vi "Google Earth.vi"() -> ()   [LabVIEW 2011]
uses:
  SubVIs/EventHandlerEnum.ctl
panel:
  in  "Tab Control":enum32{"Main", "Debug Data"}(tab)
  in  "Tilt":dbl=70.0
  in  "FPV View":bool
  in  "stop?":bool
  in  "WebBrowser":refnum<k7>(container)
  out "StreamingProgressPercentage":i32(slide) scale=0.0..100.0
  out "Camera Position 2":T1
  out "Version":string
  out "VersionAppType":i32(ring) items=["EnterpriseClientGE"=0, "ProGE"=1, "PlusGE"=2, "FreeGE"=5, "UnknownGE"=255]
  out "ElevationExaggeration":dbl
  in  "Set":bool
  in  "AutoPilotSpeed":dbl=0.5
  in  "Camera Position":T2={"Azimuth"=0.0, "FocusPointAltitude"=0.0, "altMode"=1, "FocusPointLatitude"=0.0, "FocusPointLongitude"=0.0, "Range"=0.0, "Tilt"=0.0} {"altMode" items=["RelativeToGroundAltitudeGE"=1, "AbsoluteAltitudeGE"=2]}
  in  "EARTHLib.IApplicationGE 2":refnum<k7>
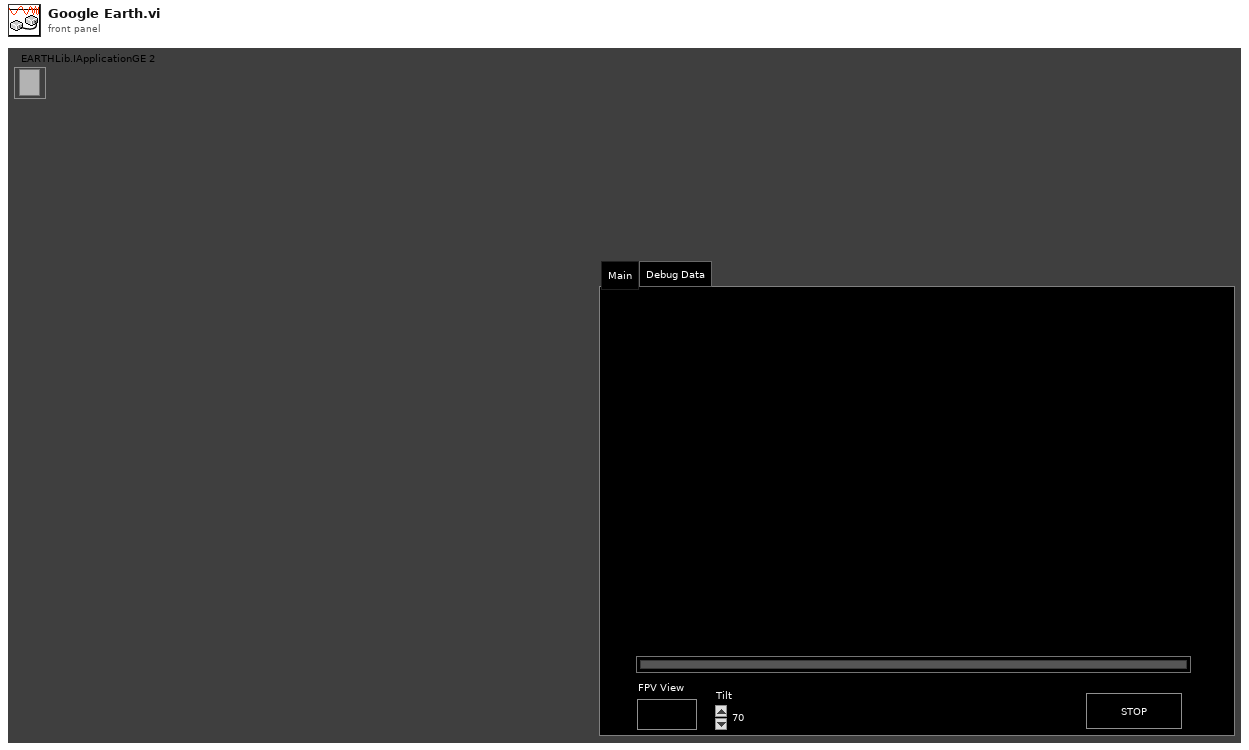
[diagram p1: front panel]
types:
  T1 = cluster{"Azimuth":dbl, "FocusPointAltitude":dbl, "FocusPointAltitudeMode":i32, "FocusPointLatitude":dbl, "FocusPointLongitude":dbl, "Range":dbl, "Tilt":dbl}
  T2 = cluster{"Azimuth":dbl, "FocusPointAltitude":dbl, "altMode":i32, "FocusPointLatitude":dbl, "FocusPointLongitude":dbl, "Range":dbl, "Tilt":dbl}
  T3 = typedef "EventHandlerEnum.ctl" = enum16{"Timeout", "Stop", "UpdateGEView", "FPV_View_On"}
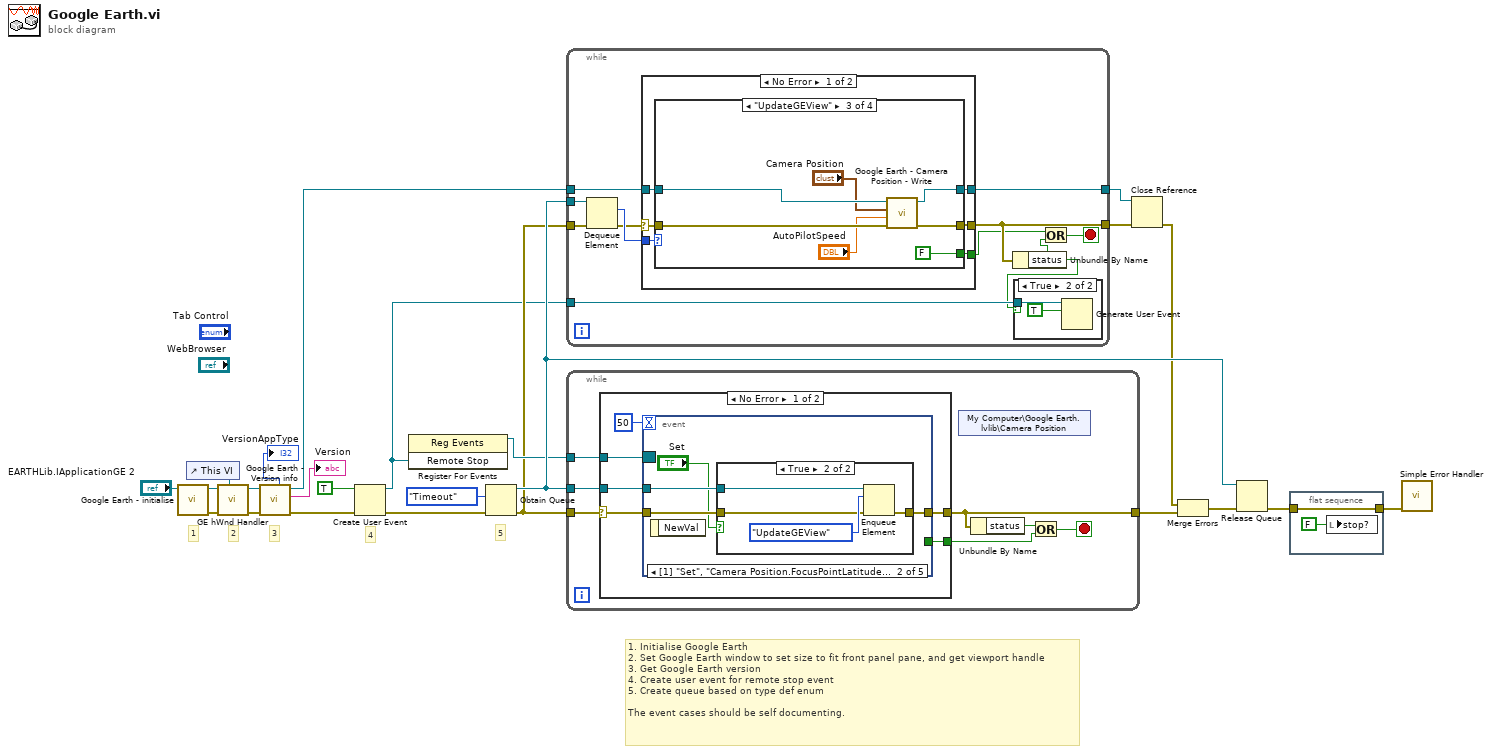
[diagram p0: block diagram]
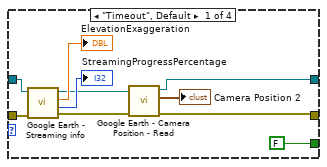
[diagram p3: hidden frame]
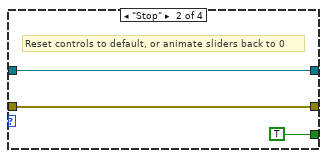
[diagram p4: hidden frame]
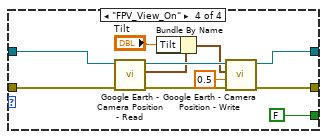
[diagram p5: hidden frame]
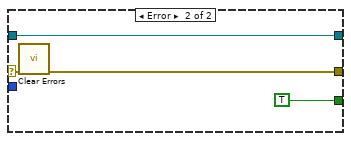
[diagram p6: hidden frame]
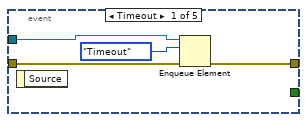
[diagram p7: hidden frame]
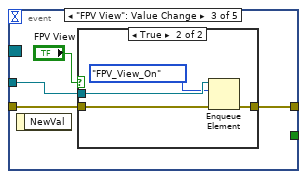
[diagram p9: hidden frame]
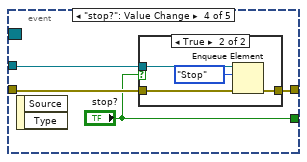
[diagram p11: hidden frame]
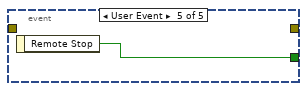
[diagram p13: hidden frame]
diagram:
  # "1. Initialise Google Earth\n2. Set Google Earth window to set size to fit front panel pane, and get viewport handle\n3. Get Google Earth version\n4. Create user event for remote stop event\n5. Create queue based on type def enum\n\nThe event cases should be self documenting."
  # "5"
  # "4"
  # "3"
  # "2"
  # "1"
  n1 = call "Google Earth - initialise.vi"("EARTHLib.IApplicationGE"="EARTHLib.IApplicationGE 2") -> ("error out"=w14:errorcluster, "Refnum Out"=w13:refnum<k7>)  [unwired: 8 in, 1 out]
  n2 = control-ref of="This VI"() -> (w21:refnum<vi>)
  n3 = call "GE hWnd Handler.vi"("This VI"=w21, "error in"=w14, "Refnum In"=w13) -> ("error out"=w22:errorcluster, "Refnum Out"=w15:refnum<k7>)  [unwired: 7 in]
  n4 = call "Google Earth - Version info.vi"("error in"=w22, "Refnum In"=w15) -> ("error out"=w2:errorcluster, "Version"=→"Version":string, "Refnum Out"=w19:refnum<k7>, "VersionAppType"=→"VersionAppType":i32)  [unwired: 6 in]
  n5 = Create User Event(user event datatype=TRUE ("Remote Stop"), error in=w2) -> (user event=w8:refnum<user-event>, error out=w12:errorcluster)
  n6 = register-events(w8) -> (reference out=w11:refnum<event-registration>)  [unwired: 2 in, 1 out]
  n7 = Obtain Queue(element data type=EventHandlerEnum."Timeout" ("Enum"), error in (no error)=w12) -> (queue out=w23:refnum<queue>, error out=w9:errorcluster)  [unwired: 3 in, 1 out]
  n8 = while {
    tunnel: w23 -> [w35]
    tunnel: [w30] -> w5
    tunnel: w19 -> [w33]
    tunnel: [w32] -> w16
    tunnel: w8 -> [w28]
    tunnel: w9 -> [w26]
    stop <- w27 stop-if-true
    n9 = Dequeue Element(queue=w35, error in (no error)=w26) -> (element=w34:T3, error out=w31:errorcluster)  [unwired: 1 in, 2 out]
    n10 = case shown="No Error" w31 {
      selector: w31 -> [w41 w78]
      tunnel: w34 -> [w43 _]
      tunnel: w33 -> [w42 w77]
      tunnel: [w40 w76] -> w30
      tunnel: [w39 w77] -> w32
      tunnel: [w38 TRUE ("x")] -> w29
      frame No Error {
        n11 = case shown="\"UpdateGEView\"" w43 {
          tunnel: w42 -> [w51 w56 w63 w72]
          tunnel: w41 -> [w45 w55 w62 w74]
          tunnel: [w46 w55 w60 w73] -> w40
          tunnel: [w48 w56 w59 w70] -> w39
          tunnel: [FALSE ("x") TRUE ("x") FALSE ("x") FALSE ("x")] -> w38
          frame "Timeout", Default {
            n12 = call "Google Earth - Streaming info.vi"("error in"=w45, "Refnum in"=w51) -> ("error out"=w47:errorcluster, "StreamingProgressPercentage"=→"StreamingProgressPercentage":i32, "ElevationExaggeration"=→"ElevationExaggeration":dbl, "Refnum Out"=w49:refnum<k7>)  [unwired: 5 in, 1 out]
            n13 = call "Google Earth - Camera Position - Read.vi"("error in"=w47, "Refnum in"=w49) -> ("error out"=w46:errorcluster, "Camera Position"=→"Camera Position 2":T1, "Refnum Out"=w48:refnum<k7>)  [unwired: 7 in]
          }
          frame "Stop" {
            # "Reset controls to default, or animate sliders back to 0"
          }
          frame "UpdateGEView" {
            n14 = call "Google Earth - Camera Position - Write.vi"("error in"=w62, "speed"="AutoPilotSpeed", "Camera Position"="Camera Position", "Refnum in"=w63) -> ("error out"=w60:errorcluster, "Refnum Out"=w59:refnum<k7>)  [unwired: 6 in]
          }
          frame "FPV_View_On" {
            n15 = call "Google Earth - Camera Position - Read.vi"("error in"=w74, "Refnum in"=w72) -> ("error out"=w66:errorcluster, "Camera Position"=w67:T1, "Refnum Out"=w71:refnum<k7>)  [unwired: 7 in]
            n16 = Bundle By Name(cluster=w67, "Tilt"="Tilt") -> (w68:T1)
            n17 = call "Google Earth - Camera Position - Write.vi"("error in"=w66, "speed"=0.5, "Camera Position"=w68, "Refnum in"=w71) -> ("error out"=w73:errorcluster, "Refnum Out"=w70:refnum<k7>)  [unwired: 6 in]
          }
        }
      }
      frame Error {
        n18 = call <vilib>:"Clear Errors.vi"("error in (no error)"=w78) -> ("error out"=w76:errorcluster)  [unwired: 6 in]
      }
    }
    n19 = Unbundle By Name(w30) -> ("status"=w25:bool)
    n20 = case shown="True" w25 {
      tunnel: w28 -> [_ w37]
      frame False {
      }
      frame True {
        n21 = Generate User Event(user event=w37, event data cluster=TRUE ("event data")) -> ()  [unwired: 1 in, 2 out]
      }
    }
    n22 = Or(x=w29, y=w25) -> (x .or. y?=w27:bool)
  }
  n23 = while {
    tunnel: w23 -> [w85]
    tunnel: w9 -> [w80]
    tunnel: [w83] -> w7
    tunnel: w11 -> [w79]
    stop <- w81 stop-if-true
    n24 = case shown="No Error" w80 {
      selector: w80 -> [w87 w124]
      tunnel: w85 -> [w91 _]
      tunnel: [w89 w124] -> w83
      tunnel: [w88 _] -> w82
      tunnel: w79 -> [w86 _]
      frame No Error {
        n25 = event shown="[1] \"Set\", \"Camera Position.FocusPointLatitude\", \"Camera Position.FocusPointLongitude\": Value Change" {
          selector: w86 -> [_ _ _ _ _]
          dyn-events: _ -> [_ _ _ _ _]
          timeout: 50 -> [_ _ _ _ _]
          tunnel: w91 -> [w95 w98 w105 w115 _]
          tunnel: w87 -> [w94 w99 w107 w117 _]
          tunnel: [w93 w97 w106 w116 _] -> w89
          tunnel: [_ _ _ "stop?" w123] -> w88
          event Timeout {
            n26 = event-data() -> ()  [unwired: 1 in, 1 out]
            n27 = Enqueue Element(queue=w95, element=EventHandlerEnum."Timeout", error in (no error)=w94) -> (error out=w93:errorcluster)  [unwired: 1 in, 2 out]
          }
          event "Set", "Camera Position.FocusPointLatitude", "Camera Position.FocusPointLongitude": Value Change {
            n28 = event-data() -> ()  [unwired: 1 in, 1 out]
            n29 = case shown="True" "Set" {
              tunnel: w99 -> [w100 w103]
              tunnel: w98 -> [_ w101]
              tunnel: [w100 w102] -> w97
              frame False {
              }
              frame True {
                n30 = Enqueue Element(queue=w101, element=EventHandlerEnum."UpdateGEView", error in (no error)=w103) -> (error out=w102:errorcluster)  [unwired: 1 in, 2 out]
              }
            }
          }
          event "FPV View": Value Change {
            n31 = event-data() -> ()  [unwired: 1 in, 1 out]
            n32 = case shown="True" "FPV View" {
              tunnel: w107 -> [w109 w113]
              tunnel: [w109 w112] -> w106
              tunnel: w105 -> [_ w111]
              frame False {
              }
              frame True {
                n33 = Enqueue Element(queue=w111, element=EventHandlerEnum."FPV_View_On", error in (no error)=w113) -> (error out=w112:errorcluster)  [unwired: 1 in, 2 out]
              }
            }
          }
          event "stop?": Value Change {
            n34 = event-data() -> ()  [unwired: 1 in, 2 out]
            n35 = case shown="True" "stop?" {
              tunnel: w117 -> [w118 w122]
              tunnel: [w118 w121] -> w116
              tunnel: w115 -> [_ w120]
              frame False {
              }
              frame True {
                n36 = Enqueue Element(queue=w120, element=EventHandlerEnum."Stop", error in (no error)=w122) -> (error out=w121:errorcluster)  [unwired: 1 in, 2 out]
              }
            }
          }
          event User Event {
            n37 = event-data() -> ("Remote Stop"=w123:bool)  [unwired: 1 in]
          }
        }
      }
      frame Error {
      }
    }
    n38 = shared-variable "My Computer\\Google Earth.lvlib\\Camera Position"() -> ()  [unwired: 1 in, 2 out]
    n39 = Unbundle By Name(w83) -> ("status"=w84:bool)
    n40 = Or(x=w84, y=w82) -> (x .or. y?=w81:bool)
  }
  n41 = Close Reference(reference=w16, error in (no error)=w5) -> (error out=w4:errorcluster)
  n42 = Merge Errors(w4, w7) -> (w6:errorcluster)
  n43 = Release Queue(queue=w23, error in (no error)=w6) -> (error out=w1:errorcluster)  [unwired: 1 in, 2 out]
  n44 = flat-sequence {
    tunnel: [w125] -> w3
    tunnel: w1 -> [w125]
    frame #0 {
      n45 = local write "stop?"(FALSE ("Stop")) -> ()
    }
  }
  n46 = call <vilib>:"Simple Error Handler.vi"("error in (no error)"=w3) -> ()  [unwired: 4 in, 5 out]
